vi "load_user_data.vi"(8 "error in (no error)":errorcluster, 10 "sections":string[](array[string]), 11 "file_name":string) -> (0 "error out":errorcluster, 3 "user settings":string[][](array[string]))   [LabVIEW 2024]
uses:
  <vilib>/Utility/config.llb/Read Key (String).vi
  <vilib>/Utility/config.llb/NI_LVConfig.lvlib
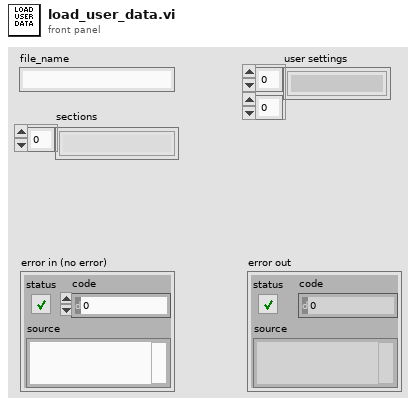
[diagram p1: front panel]
types:
  T1 = typedef "NI_LVConfig.lvlib/Config Data RefNum.ctl" = refnum<k1>
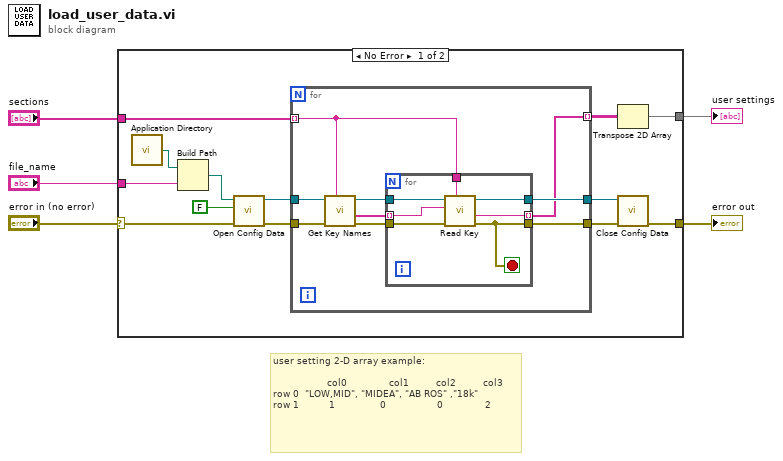
[diagram p0: block diagram]
diagram:
  # "user setting 2-D array example:\n\n                  col0              col1         col2         col3\nrow 0  \"LOW,MID\", \"MIDEA\", \"AB ROS\" ,\"18k\" \nrow 1          1               0                 0              2"
  n1 = case shown="No Error" "error in (no error)" {
    selector: "error in (no error)" -> [w9 w35]
    tunnel: [w17 w35] -> w5
    tunnel: "file_name" -> [w11 _]
    tunnel: "sections" -> [w8 _]
    tunnel: [w6 _] -> w1
    frame No Error {
      n2 = call <vilib>:"Application Directory.vi"() -> ("Application Directory"=w10:path)
      n3 = Build Path(base path=w10, name or relative path=w11) -> (appended path=w18:path)
      n4 = call <vilib>:"Open Config Data.vi"("error in (no error)"=w9, "create file if necessary (T)"=FALSE, "configuration file path"=w18) -> ("error out"=w14:errorcluster, "refnum"=w13:T1)  [unwired: 6 in, 1 out]
      n5 = for {
        tunnel: w8 -> [w20] mode=indexing
        tunnel: w13 -> [w21]
        tunnel: [w26] -> w15
        tunnel: w14 -> [w22]
        tunnel: [w27] -> w16
        tunnel: [w19] -> w7 mode=indexing
        n6 = call <vilib>:"Get Key Names.vi"("section"=w20, "error in (no error)"=w22, "refnum"=w21) -> ("error out"=w23:errorcluster, "key names"=w25:string[], "refnum out"=w24:T1)  [unwired: 5 in, 1 out]
        n7 = for {
          tunnel: w23 -> [w34]
          tunnel: w24 -> [w33]
          tunnel: w25 -> [w29] mode=indexing
          tunnel: [w32] -> w19 mode=indexing
          tunnel: [w31] -> w27
          tunnel: [w30] -> w26
          tunnel: w20 -> [w28]
          stop <- w31 stop-if-true
          n8 = call-poly <vilib>:"Read Key.vi"("section"=w28, "error in (no error)"=w34, "key"=w29, "refnum"=w33) -> ("error out"=w31:errorcluster, "value"=w32:string, "refnum out"=w30:T1)  [unwired: 4 in, 1 out]
        }
      }
      n9 = Transpose 2D Array(2D array=w7) -> (transposed array=w6:string[][])
      n10 = call <vilib>:"Close Config Data.vi"("error in (no error)"=w16, "refnum"=w15) -> ("error out"=w17:errorcluster)  [unwired: 8 in, 1 out]
    }
    frame Error {
    }
  }
  "error out" <- w5
  "user settings" <- w1
